vi "DQMH Request Reply Timed Out--error.vi"(9 "timed out?":bool, 10 "Module Name":string, 11 "Request Name":string) -> (0 "error out":errorcluster)   [LabVIEW 2014, in "hse-dqmh.lvlib"]
uses:
  hse-dqmh.lvlib
  <vilib>/Utility/error.llb/Error Cluster From Error Code.vi
  <vilib>/ErrorRing/Error Ring.xnode
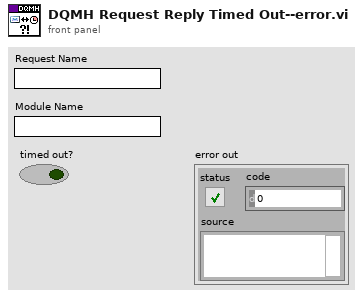
[diagram p1: front panel]
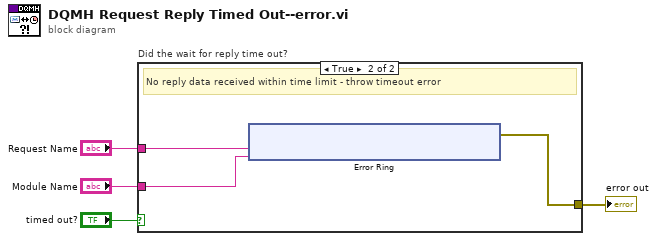
[diagram p0: block diagram]
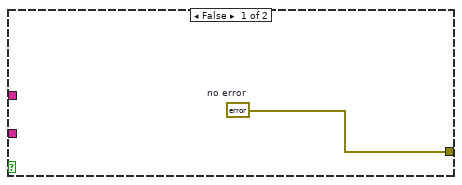
[diagram p2: hidden frame]
diagram:
  n1 = case "Did the wait for reply time out?" shown="True" "timed out?" {
    tunnel: [w5 w8] -> w3
    tunnel: "Request Name" -> [_ w7]
    tunnel: "Module Name" -> [_ w6]
    frame False {
      w5 = errorcluster {"status"=FALSE, "code"=0, "source"=""}  # no error
    }
    frame True {
      # "No reply data received within time limit - throw timeout error"
      n2 = xnode "Error Ring"("parameter 0"=w7, "parameter 1"=w6) -> ("error out"=w8:errorcluster)
    }
  }
  "error out" <- w3
